vi "UpdateSelectRing.vi"(8 "error in (no error)":errorcluster, 10 "CloneRegRef":refnum<data-value>, 11 "Ring Refnum":refnum<vi>) -> (0 "error out":errorcluster, 1 "ActiveModules":string[](array[string]), 2 "Module Ring Value":i32=-1)   [LabVIEW 2014, in "WfrmModule.lvlib"]
uses:
  WfrmModule.lvlib
  <userlib>/NIST/ModuleAdminLib/CloneRegistration/CloneRegistration.lvclass
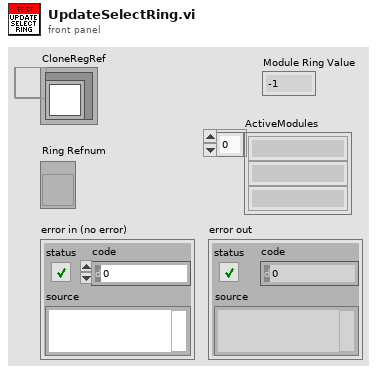
[diagram p1: front panel]
types:
  T1 = typedef "LVStringsAndValuesArrayTypeDef.ctl" = cluster{"String":string, "Value":ext}[]
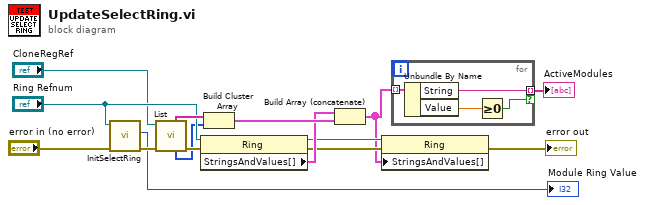
[diagram p0: block diagram]
diagram:
  n1 = call "InitSelectRing.vi"("error in (no error)"="error in (no error)", "Ring Refnum"="Ring Refnum") -> ("error out"=w14:errorcluster, "Module Ring Value"=→"Module Ring Value":i32)  [unwired: 8 in]
  n2 = call <userlib>:"List.vi"("error in (no error)"=w14, "CloneRegRef"="CloneRegRef") -> ("error out"=w12:errorcluster, "Module IDs"=w1:i32[], "Instance Names"=w13:string[])  [unwired: 4 in, 3 out]
  n3 = property class="Ring"(reference="Ring Refnum", error in=w12) -> (reference out=w8:refnum<vi>, error out=w9:errorcluster, "StringsAndValues[]"=w10:T1)
  n4 = Build Cluster Array(w13, w1) -> (w11:cluster{string, i32}[])
  n5 = Build Array (concatenate)(w10, w11) -> (w7:T1)
  n6 = property class="Ring"(reference=w8, error in=w9, "StringsAndValues[]"=w7) -> (error out=→"error out":errorcluster)  [unwired: 1 out]
  n7 = for {
    tunnel: w7 -> [w19] mode=indexing
    tunnel: [w18] -> w6 mode=indexing if=w17
    n8 = Unbundle By Name(w19) -> ("String"=w18:string, "Value"=w16:ext)
    n9 = Greater Or Equal To 0?(x=w16) -> (x >= 0?=w17:bool)
  }
  "ActiveModules" <- w6
